vi "DeviceStartupSequence.vi"(8 "error in":errorcluster) -> (0 "error out":errorcluster, 3 "DeviceStartUpDone":bool)   [LabVIEW 2011]
uses:
  Variables/GlobalGetPhysikalInstrumentsOnOff.vi
  Variables/GlobalGetKoherasLaserOnOff.vi
  Variables/GlobalGetAOTFOnOff.vi
  Variables/GlobalGetCamerasOnOff.vi
  Variables/GlobalGetInitialisationStatus.vi
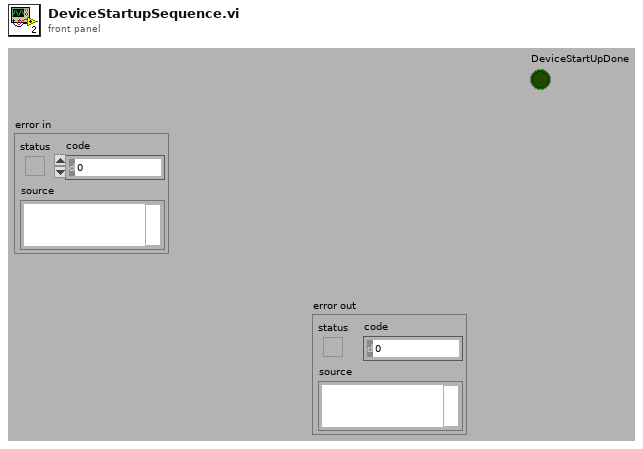
[diagram p1: front panel]
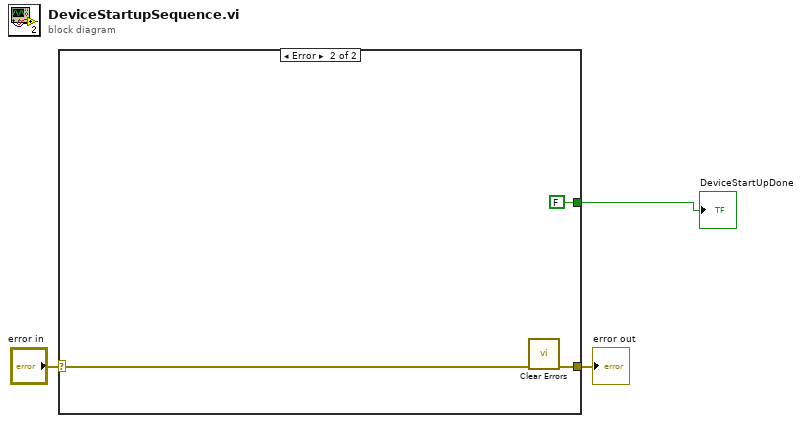
[diagram p0: block diagram]
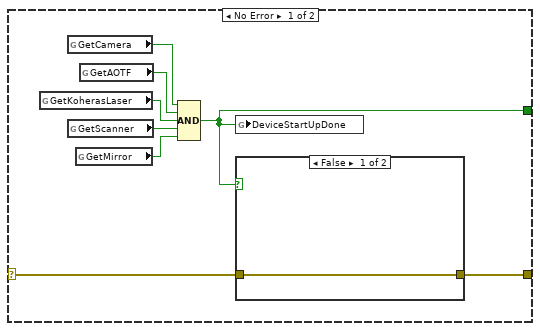
[diagram p2: hidden frame]
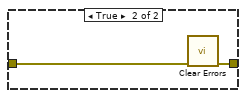
[diagram p3: hidden frame]
diagram:
  n1 = case shown="Error" "error in" {
    selector: "error in" -> [w10 w16]
    tunnel: [w11 w17] -> w2
    tunnel: [w4 FALSE] -> w1
    frame No Error {
      n2 = global read "GlobalGetKoherasLaserOnOff.vi" "GetKoherasLaser"() -> (w7:bool)
      n3 = global read "GlobalGetCamerasOnOff.vi" "GetCamera"() -> (w9:bool)
      n4 = global read "GlobalGetPhysikalInstrumentsOnOff.vi" "GetScanner"() -> (w6:bool)
      n5 = global read "GlobalGetPhysikalInstrumentsOnOff.vi" "GetMirror"() -> (w5:bool)
      n6 = global read "GlobalGetAOTFOnOff.vi" "GetAOTF"() -> (w8:bool)
      n7 = Compound Arithmetic op=AND(w9, w8, w7, w6, w5) -> (w4:bool)
      n8 = global write "GlobalGetInitialisationStatus.vi" "DeviceStartUpDone"(w4) -> ()
      n9 = case shown="False" w4 {
        tunnel: [w12 w14] -> w11
        tunnel: w10 -> [w12 w13]
        frame False {
        }
        frame True {
          n10 = call <vilib>:"Clear Errors.vi"("error in (no error)"=w13) -> ("error out"=w14:errorcluster)  [unwired: 6 in]
        }
      }
    }
    frame Error {
      n11 = call <vilib>:"Clear Errors.vi"("error in (no error)"=w16) -> ("error out"=w17:errorcluster)  [unwired: 6 in]
    }
  }
  "error out" <- w2
  "DeviceStartUpDone" <- w1
